vi "Send String.vi"(6 "error in (no error)":errorcluster, 8 "Bus In":refnum<class "Bus.lvclass">, 9 "No Init In":refnum<class "No Init.lvclass">) -> (0 "error out":errorcluster, 2 "Bus Out":refnum<class "Bus.lvclass">, 3 "No Init out":refnum<class "No Init.lvclass">)   [LabVIEW 2018, in "No Init.lvclass"]
doc: "No Init.lvclass:Send String.vi\n\nThis is the Send String VI for No Init.\nInstrument Communication Module Version 1.0\nOctober, 2020 Original Code Consulting Davita Bird\n www.originalcode.com"
uses:
  No Init.lvclass
  Bus/Bus.lvclass
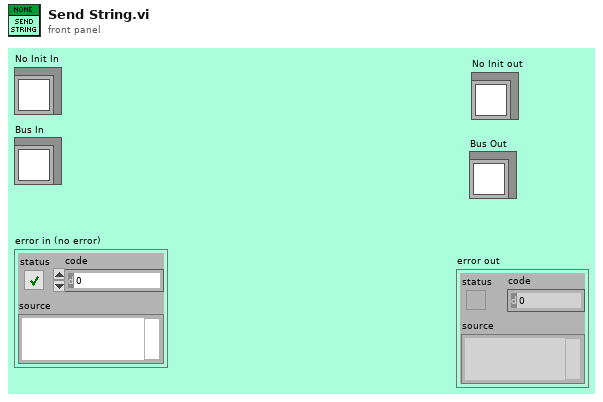
[diagram p1: front panel]
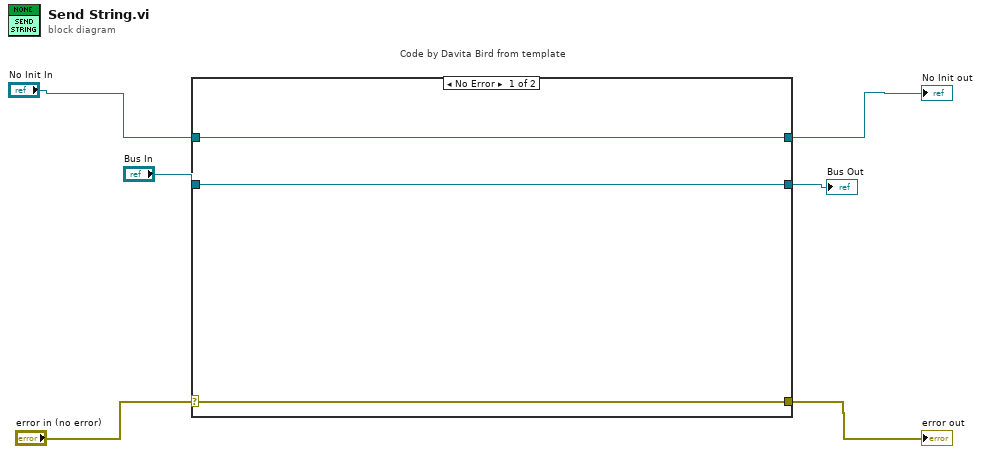
[diagram p0: block diagram]
diagram:
  n1 = case "Code by Davita Bird from template" shown="No Error" "error in (no error)" {
    selector: "error in (no error)" -> [w8 w12]
    tunnel: [w8 w12] -> w1
    tunnel: [w9 w11] -> w5
    tunnel: "No Init In" -> [w9 w11]
    tunnel: [w7 w10] -> w3
    tunnel: "Bus In" -> [w7 w10]
    frame No Error {
    }
    frame Error {
    }
  }
  "error out" <- w1
  "No Init out" <- w5
  "Bus Out" <- w3
